vi "Sample And Hold.vi"(10 "Signal":dbl, 11 "Condition":bool) -> (3 "Signal Out":dbl)   [LabVIEW 2015]
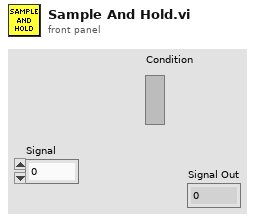
[diagram p1: front panel]
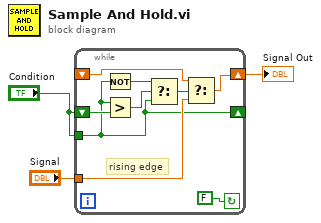
[diagram p0: block diagram]
diagram:
  n1 = while {
    tunnel: "Signal" -> [w11]
    shift-right: [w10] -> w2
    shift-left: _ -> [w9]
    shift-right: [w4] -> _
    shift-left: "Condition" -> [w8]
    tunnel: "Condition" -> [w4]
    stop <- FALSE continue-if-true
    # "rising edge"
    n2 = Not(x=w4) -> (.not. x?=w6:bool)
    n3 = Greater?(x=w4, y=w8) -> (0:w7:bool)
    n4 = Select(t=w6, s=w7, f=w4) -> (s? t:f=w5:bool)
    n5 = Select(t=w9, s=w5, f=w11) -> (s? t:f=w10:dbl)
  }
  "Signal Out" <- w2
